vi "main_FGV.vi"(7 "Mode":T1, 8 "error in":errorcluster, 11 "Parameter in":variant) -> (0 "error out":errorcluster, 3 "Parameter out":variant)   [LabVIEW 2016]
uses:
  modes_mains_FGV.ctl
  cluster_main_FGV.ctl
  Config/Channel_config.ctl
  Config/test_config.ctl
  Config/feedType.ctl
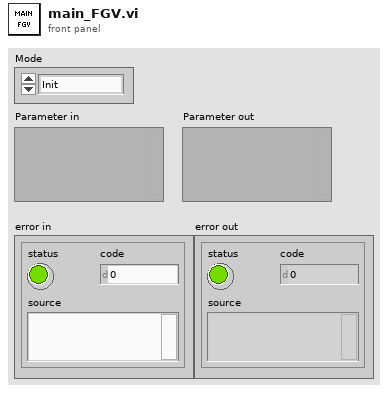
[diagram p1: front panel]
types:
  T1 = typedef "modes_mains_FGV.ctl" = enum16{"Init", "Config", "CreateDir", "CreateTask", "CreateQueues", "Record", "Comment", "GetFeed", "GetInc", "End"}
  T2 = typedef "cluster_main_FGV.ctl" = cluster{"Simulation?":bool, "ChanConfigs":T3[], "Test Config":T4, "Directory":path, "TestName":string, "RawFile":refnum<file>, "InfoFile":refnum<file>, "DataFile":refnum<file>, "task":refnum<k21>, "qRecord":refnum<queue>, "qProcess":refnum<queue>, "feed":T5}
  T3 = typedef "Channel_config.ctl" = cluster{"Canal":i32, "GF":dbl, "SC":bool}
  T4 = typedef "test_config.ctl" = cluster{"HoleDiam":dbl, "MeanLineDiam":dbl, "IncF":dbl, "ElastMod":dbl, "PoissonMod":dbl, "RosType":enum16{"Tipo A", "Tipo B", "Tipo C"}, "Método de análise":enum16{"Não uniforme 2013", "Simplificado 2013", "Simplificado 2008"}, "Pfinal":dbl, "AStop":bool}
  T5 = typedef "feedType.ctl" = enum16{"Manual", "Automático"}
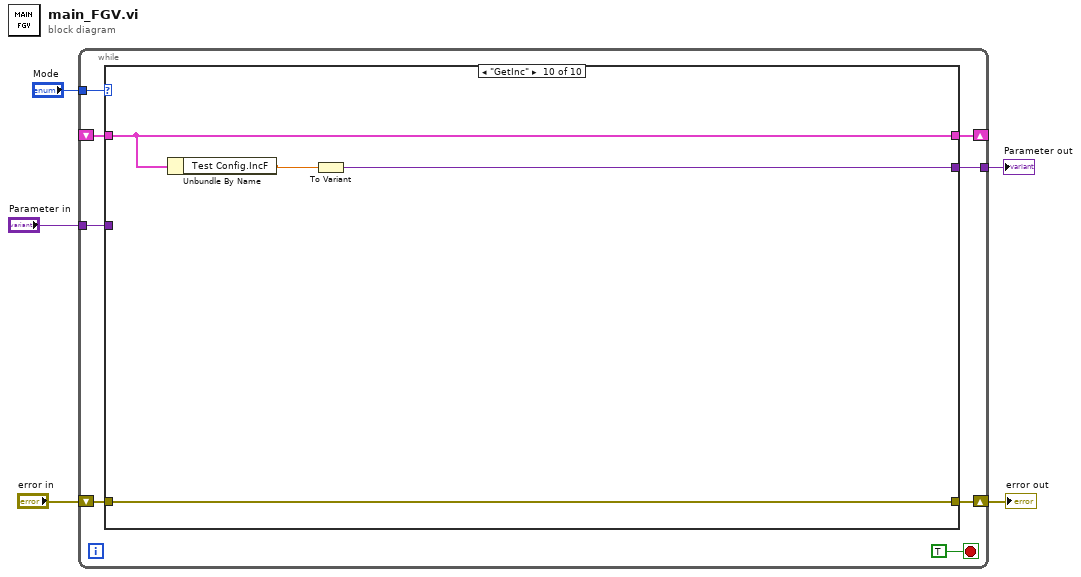
[diagram p0: block diagram]
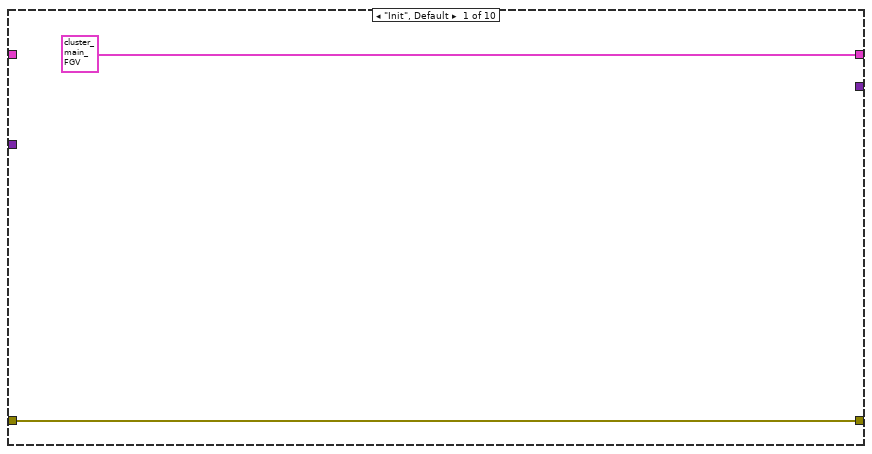
[diagram p2: hidden frame]
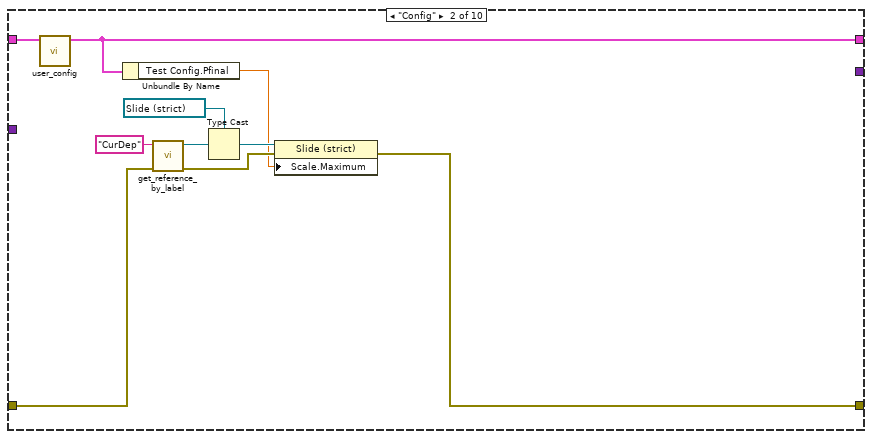
[diagram p3: hidden frame]
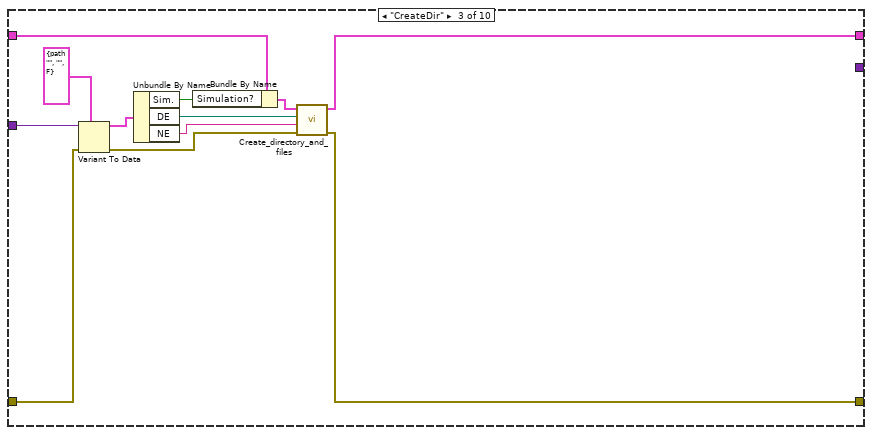
[diagram p4: hidden frame]
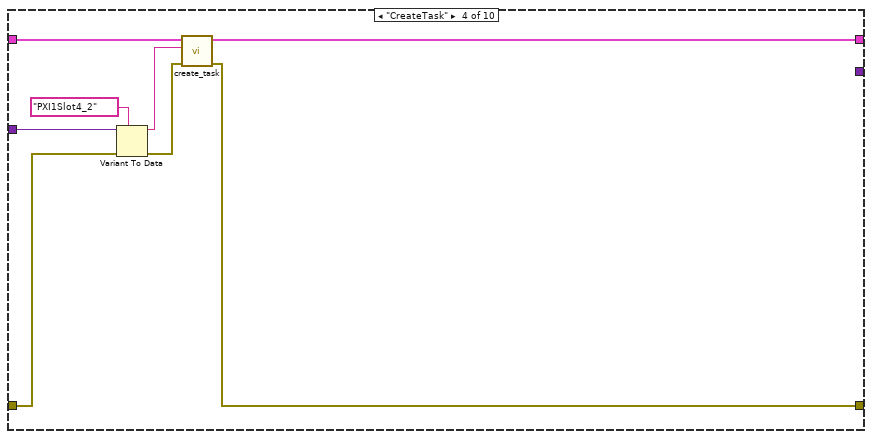
[diagram p5: hidden frame]
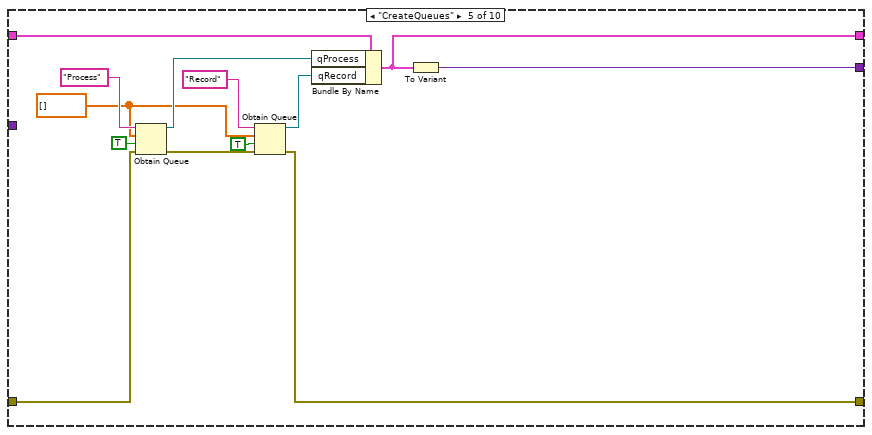
[diagram p6: hidden frame]
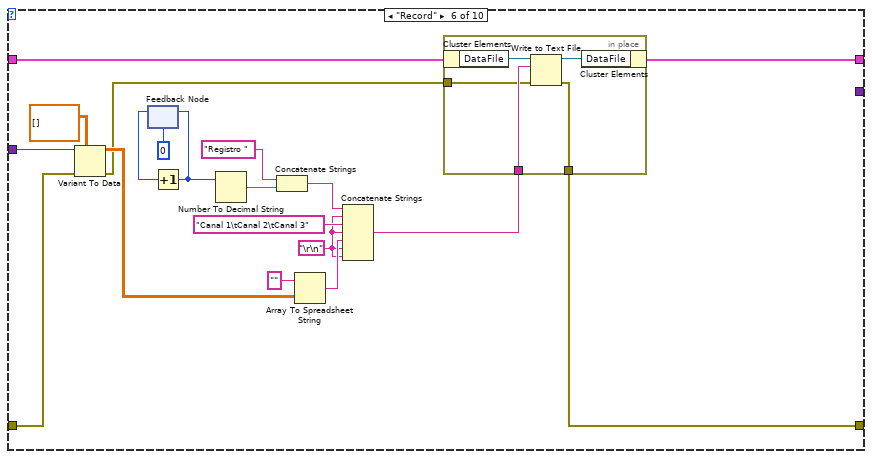
[diagram p7: hidden frame]
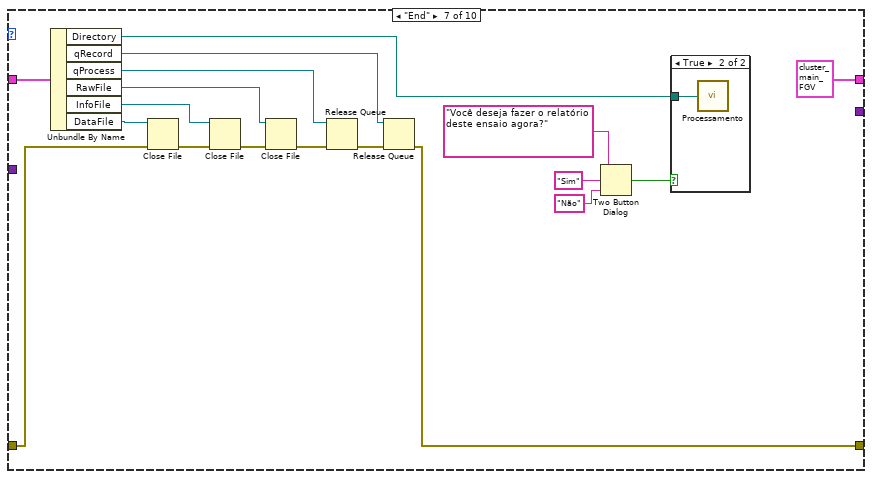
[diagram p8: hidden frame]
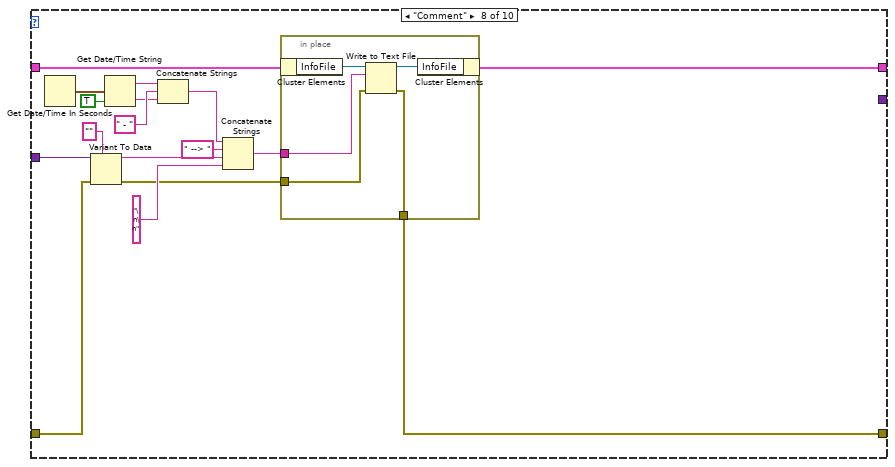
[diagram p10: hidden frame]
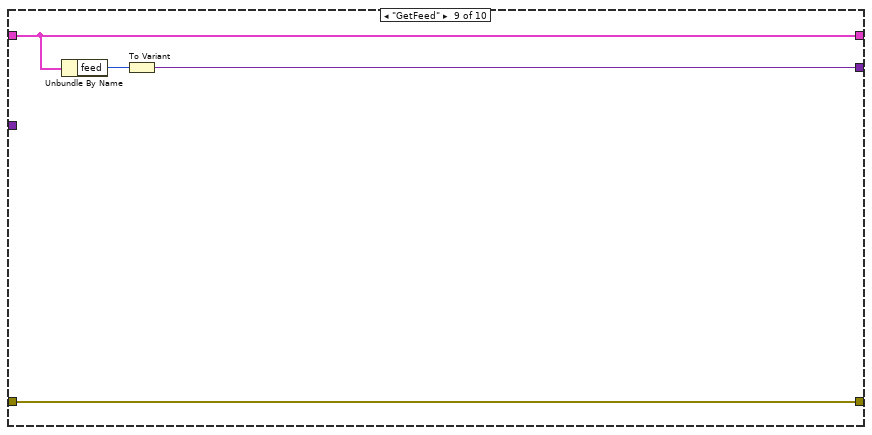
[diagram p11: hidden frame]
diagram:
  n1 = while {
    tunnel: "Mode" -> [w12]
    shift-right: [w11] -> _
    shift-left: _ -> [w8]
    shift-right: [w9] -> w3
    shift-left: "error in" -> [w10]
    tunnel: "Parameter in" -> [w7]
    tunnel: [w6] -> w1
    stop <- TRUE stop-if-true
    n2 = case shown="\"GetInc\"" w12 {
      tunnel: [T2 {"Simulation?"=FALSE, "ChanConfigs"=[], "Test Config"={"HoleDiam"=1.4, "MeanLineDiam"=5.0, "IncF"=0.2, "ElastMod"=207.0, "PoissonMod"=0.3, "RosType"=enum."Tipo A", "Método de análise"=enum."Simplificado 2008", "Pfinal"=0.3, "AStop"=TRUE}, "Directory"=path "", "TestName"="", "RawFile"=refnum, "InfoFile"=refnum, "DataFile"=refnum, "task"="", "qRecord"=refnum, "qProcess"=refnum, "feed"=enum."Manual"} ("cluster_main_FGV") w18 w32 w38 w51 w59 T2 {"Simulation?"=FALSE, "ChanConfigs"=[], "Test Config"={"HoleDiam"=1.4, "MeanLineDiam"=5.0, "IncF"=0.2, "ElastMod"=207.0, "PoissonMod"=0.3, "RosType"=enum."Tipo A", "Método de análise"=enum."Simplificado 2008", "Pfinal"=0.3, "AStop"=TRUE}, "Directory"=path "", "TestName"="", "RawFile"=refnum, "InfoFile"=refnum, "DataFile"=refnum, "task"="", "qRecord"=refnum, "qProcess"=refnum, "feed"=enum."Manual"} ("Cluster") w109 w126 w130] -> w11
      tunnel: w10 -> [w14 w24 w36 w42 w49 w64 w98 w117 w125 w129]
      tunnel: [w14 w16 w30 w39 w52 w60 w88 w110 w125 w129] -> w9
      tunnel: w8 -> [_ w25 w28 w45 w48 w62 w99 w115 w126 w130]
      tunnel: w7 -> [_ _ w37 w44 _ w66 _ w118 _ _]
      tunnel: [_ _ _ _ w50 _ _ _ w124 w128] -> w6
      frame "Init", Default {
      }
      frame "Config" {
        n3 = call "user_config.vi"("ClusterIn"=w25) -> ("ClusterOut"=w18:T2)  [unwired: 10 in]
        n4 = Unbundle By Name(w18) -> ("Test Config.Pfinal"=w17:dbl)
        n5 = call "get_reference_by_label.vi"("error in"=w24, "Label"="CurDep") -> ("error out"=w19:errorcluster, "Ctl Refnum"=w22:refnum<vi>)  [unwired: 7 in, 1 out]
        n6 = Type Cast(type=refnum<vi> refnum ("CurrentDepth"), x=w22) -> (*(type *) &x=w20:refnum<vi>)
        n7 = property on="Property Node" class="Slide (strict)"(reference=w20, error in=w19, "Scale.Maximum"=w17) -> (error out=w16:errorcluster)  [unwired: 1 out]
      }
      frame "CreateDir" {
        n8 = Variant To Data(error in=w36, type=cluster{"DE":path, "NE":string, "Sim.":bool} {"DE"=path "", "NE"="", "Sim."=FALSE} ("output cluster"), Variant=w37) -> (data=w35:cluster{"DE":path, "NE":string, "Sim.":bool}, error out=w31:errorcluster)
        n9 = Unbundle By Name(w35) -> ("Sim."=w27:bool, "DE"=w34:path, "NE"=w33:string)
        n10 = Bundle By Name(cluster=w28, "Simulation?"=w27) -> (w26:T2)
        n11 = call "Create_directory_and_files.vi"("error in"=w31, "NE"=w33, "DE"=w34, "ClusterIn"=w26) -> ("error out"=w30:errorcluster, "ClusterOut"=w32:T2)  [unwired: 6 in]
      }
      frame "CreateTask" {
        n12 = Variant To Data(error in=w42, type=tag "PXI1Slot4_2" ("NP"), Variant=w44) -> (data=w40:tag, error out=w41:errorcluster)
        n13 = call "create_task.vi"("error in"=w41, "NP"=w40, "ClusterIn"=w45) -> ("error out"=w39:errorcluster, "Cluster"=w38:T2)  [unwired: 7 in]
      }
      frame "CreateQueues" {
        w46 = dbl[] [] ("2D array")
        n14 = Obtain Queue(name (unnamed)="Process", element data type=w46, create if not found? (T)=TRUE, error in (no error)=w49) -> (queue out=w47:refnum<queue>, error out=w54:errorcluster)  [unwired: 1 in, 1 out]
        n15 = Obtain Queue(name (unnamed)="Record", element data type=w46, create if not found? (T)=TRUE, error in (no error)=w54) -> (queue out=w53:refnum<queue>, error out=w52:errorcluster)  [unwired: 1 in, 1 out]
        n16 = Bundle By Name(cluster=w48, "qProcess"=w47, "qRecord"=w53) -> (w51:T2)
        n17 = To Variant(anything=w51) -> (Variant=w50:variant)
      }
      frame "Record" {
        w71 = "\r\n"
        n18 = Variant To Data(error in=w64, type=dbl[][] [] ("Dados"), Variant=w66) -> (data=w63:dbl[][], error out=w61:errorcluster)
        n19 = feedback #1(0) -> (w69:i32)
        n20 = Increment(x=w69) -> (x+1=w67:i32)
        n21 = feedback-in #1(w67) -> ()
        n22 = Number To Decimal String(number=w67) -> (decimal integer string=w73:string)  [unwired: 1 in]
        n23 = Concatenate Strings("Registro " ("string"), w73) -> (w72:string)
        n24 = Array To Spreadsheet String(array=w63, 3:"" ("format string")) -> (spreadsheet string=w75:string)  [unwired: 1 in]
        n25 = Concatenate Strings(w72, w71, "Canal 1\tCanal 2\tCanal 3", w71, w75, w71, w71) -> (w70:string)
        n26 = in-place {
          in-place-border: w70 -> [w82]
          in-place-border: w61 -> [w79]
          in-place-border: [w78] -> w60
          n27 = in-place-cluster #2(w62) -> ("DataFile"=w81:refnum<file>)
          n28 = Write to Text File(file (use dialog)=w81, text=w82, error in=w79) -> (refnum out=w80:refnum<file>, error out=w78:errorcluster)  [unwired: 1 in, 1 out]
          n29 = in-place-cluster #2("DataFile"=w80) -> (w59:T2)
        }
      }
      frame "End" {
        n30 = Unbundle By Name(w99) -> ("Directory"=w83:path, "qRecord"=w89:refnum<queue>, "qProcess"=w91:refnum<queue>, "RawFile"=w93:refnum<file>, "InfoFile"=w95:refnum<file>, "DataFile"=w97:refnum<file>)
        n31 = Close File(refnum=w97, error in=w98) -> (error out=w96:errorcluster)  [unwired: 1 out]
        n32 = Close File(refnum=w95, error in=w96) -> (error out=w94:errorcluster)  [unwired: 1 out]
        n33 = Close File(refnum=w93, error in=w94) -> (error out=w92:errorcluster)  [unwired: 1 out]
        n34 = Release Queue(queue=w91, error in (no error)=w92) -> (error out=w90:errorcluster)  [unwired: 1 in, 2 out]
        n35 = Release Queue(queue=w89, error in (no error)=w90) -> (error out=w88:errorcluster)  [unwired: 1 in, 2 out]
        n36 = Two Button Dialog(message="Você deseja fazer o relatório deste ensaio agora?", 1:"Não" ("F button name (\"Cancel\")"), 2:"Sim" ("T button name (\"OK\")")) -> (T button?=w84:bool)
        n37 = case shown="True" w84 {
          tunnel: w83 -> [_ w101]
          frame False {
          }
          frame True {
            n38 = call "Processamento.vi"("Pasta do ensaio"=w101) -> ()
          }
        }
      }
      frame "Comment" {
        n39 = Get Date/Time In Seconds() -> (seconds since 1Jan1904=w108:timestamp)
        n40 = Variant To Data(error in=w117, type="" ("name (unnamed)"), Variant=w118) -> (data=w114:string, error out=w112:errorcluster)
        n41 = Get Date/Time String(seconds (now)=w108, want seconds? (F)=TRUE) -> (date string=w106:string, time string=w104:string)  [unwired: 1 in]
        n42 = Concatenate Strings(w106, " - " ("string"), w104) -> (w103:string)
        n43 = Concatenate Strings(w103, " --> " ("string"), w114, "\n\n" ("string")) -> (w111:string)
        n44 = in-place {
          in-place-border: w112 -> [w121]
          in-place-border: w111 -> [w120]
          in-place-border: [w119] -> w110
          n45 = in-place-cluster #3(w115) -> ("InfoFile"=w123:refnum<file>)
          n46 = Write to Text File(file (use dialog)=w123, text=w120, error in=w121) -> (refnum out=w122:refnum<file>, error out=w119:errorcluster)  [unwired: 1 in, 1 out]
          n47 = in-place-cluster #3("InfoFile"=w122) -> (w109:T2)
        }
      }
      frame "GetFeed" {
        n48 = Unbundle By Name(w126) -> ("feed"=w127:T5)
        n49 = To Variant(anything=w127) -> (Variant=w124:variant)
      }
      frame "GetInc" {
        n50 = Unbundle By Name(w130) -> ("Test Config.IncF"=w131:dbl)
        n51 = To Variant(anything=w131) -> (Variant=w128:variant)
      }
    }
  }
  "error out" <- w3
  "Parameter out" <- w1
